vi "RFSoC_test.vi"() -> ()   [LabVIEW 2019]
uses:
  Pulse Parameters.ctl
  RFSoC Driver.lvclass
  C:/GitHub/NHMFL_Core/Libraries/Instruments/RFSoC/2019/GitHub/NHMFL_Core/Libraries/Instruments/Pulse Driver/Pulse Driver.lvclass
  RFSoC Driver.lvclass/RFSoC Driver.ctl
  Pulse Driver/Pulse Driver.lvclass/Pulse Driver.ctl
  Utilities/Output Value/Output Value.lvclass
  C:/GitHub/NHMFL_Core/Libraries/Instruments/RFSoC/2019/GitHub/NHMFL_Core/Libraries/Instruments/Results/Acquired Result/Acquired Result.lvclass
  Write address.vi
  Pulse Driver/Write Samples per read.vi
  Pulse Driver/Write Binary sample width.vi
  Write Mixer.vi
panel:
  in  "Mixer":enum16{"Real", "I/Q"}(ring)=enum."I/Q"
  in  "Samples per read":i32=8192
  in  "Tab Control":enum32{"Page 1", "Page 2"}(tab)
  in  "Send Button":bool
  out "Manual responce":string
  in  "Manual command":string
  in  "Initial commands SSR":string[](array[string])=["SetMemType 0", "SetBitstream 3", "MultiBand 0 0 0x1 0x2 0x1", "MultiBand 0 0 0x2 0x2 0x2", "SetMixerSettings 0 0 0 0.000000 0.000000 2 1 16 4 0", "UpdateEvent 0 0 0 1", "SetupFIFO 0 0 0", "SetDecimationFactor 0 0 1", "SetFabClkOutDiv 0 0 2", "IntrClr 0 0 0 0xFFFFFFFF", "SetupFIFO 0 0 1"]
  in  "Initial commands":string[](array[string])=["SetBitstream 1", "MultiBand 0 0 0x1 0x2 0x1", "MultiBand 0 0 0x2 0x2 0x2", "SetMixerSettings 0 0 0 -190.000000 0.000000 2 2 0 3 0", "UpdateEvent 0 0 0 1", "SetupFIFO 0 0 0", "SetDecimationFactor 0 0 1", "SetFabClkOutDiv 0 0 2", "IntrClr 0 0 0 0xFFFFFFFF", "SetupFIFO 0 0 1"]
  out "Responce":string[](array[string])
  out "Record responce":string[](array[string])
  in  "Generate commands 1":string[](array[string])=["LocalMemInfo 1", "LocalMemTrigger 1 0 0 0x0000"]
  in  "Generate commands 2":string[](array[string])=["SetLocalMemSample 1 1 3 8192", "LocalMemTrigger 1 1 0 0x0080", "LocalMemInfo 1"]
  out "Waveform Graph":cluster{dbl, dbl, dbl[][]}(graph)
  in  "Pulse Parameters":T1={"clock rate"=6389760000.0, "Frequency"=217000000.0, "NWaves"=75, "standard deviation"=0.1, "Amplitude"=30000.0, "Mode"=enum."Pulse"} {"Frequency" format="%#_6pHz"; "clock rate" format="%#_6pHz"}
  in  "Generate Button":bool
  in  "Output frequency":dbl=2000000.0 format="%#_6pHz"
  in  "Record  Button":bool
  out "FW Version":string
  in  "Stop Button":bool
  in  "address":string="192.168.1.3"
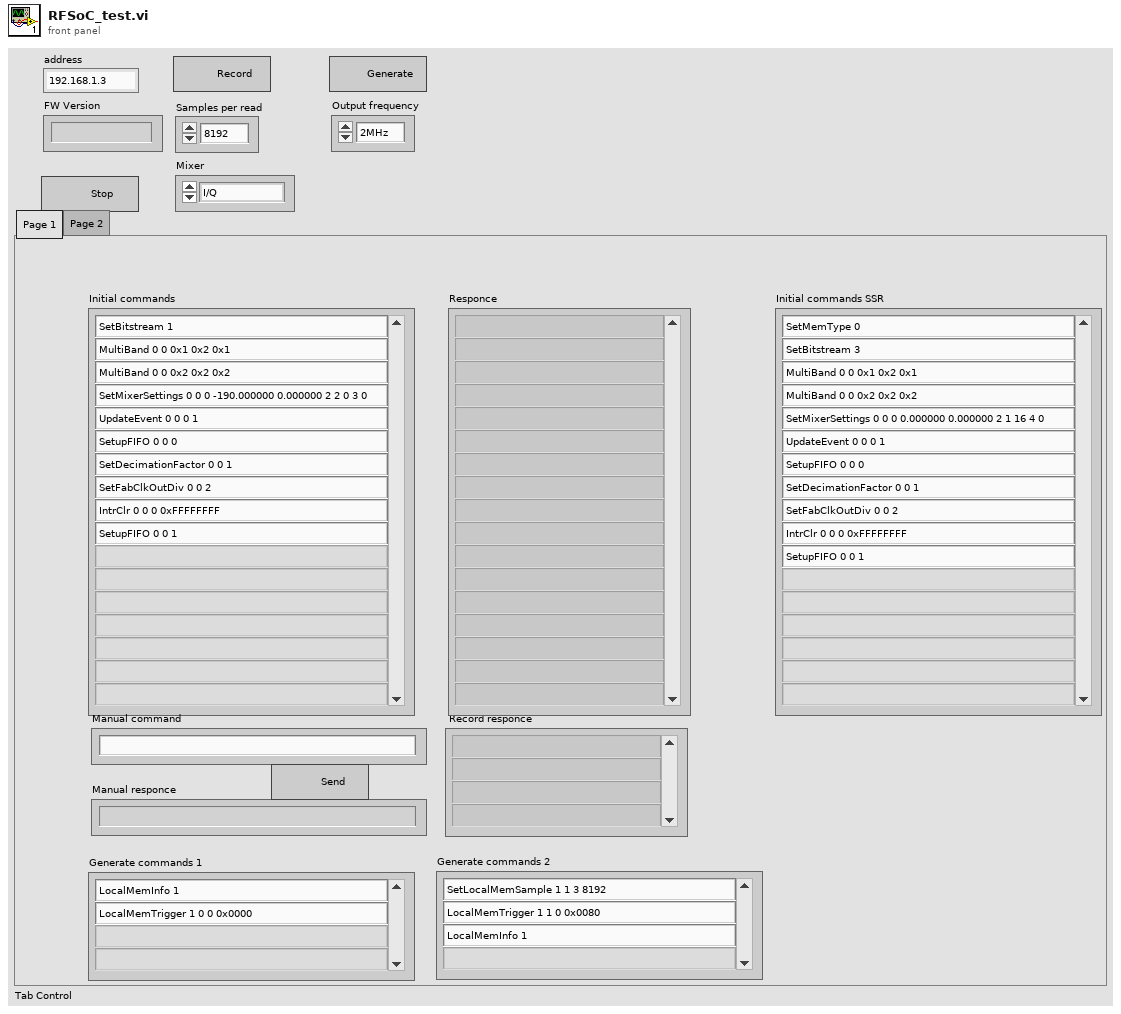
[diagram p1: front panel]
types:
  T1 = typedef "Pulse Parameters.ctl" = cluster{"clock rate":dbl, "Frequency":dbl, "NWaves":i32, "standard deviation":dbl, "Amplitude":dbl, "Mode":enum16{"Sine", "Pulse"}}
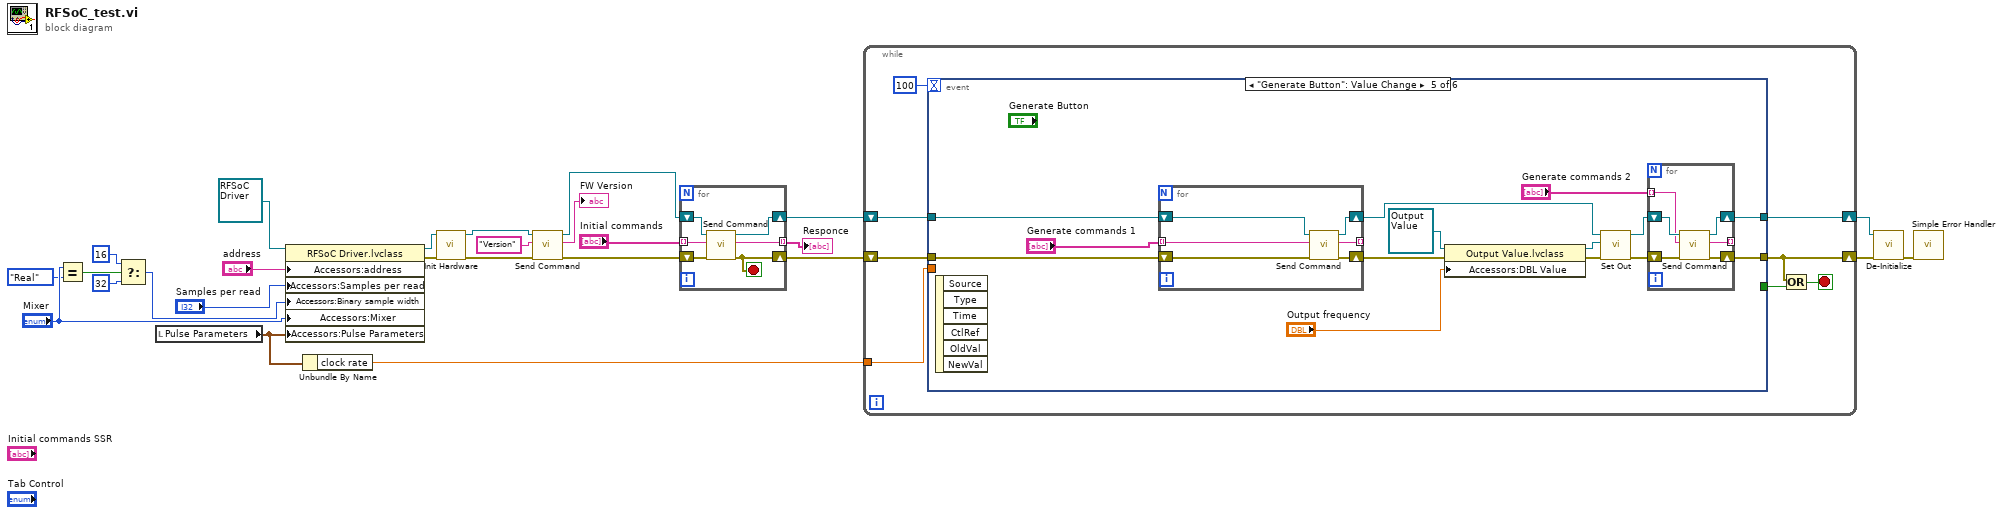
[diagram p0: block diagram]
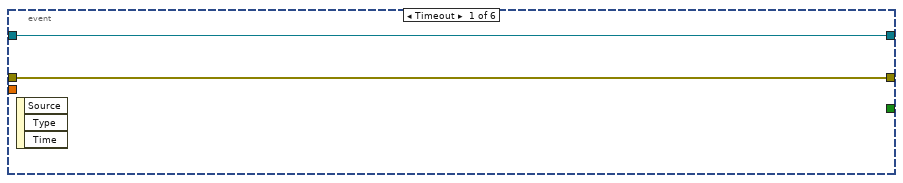
[diagram p2: hidden frame]
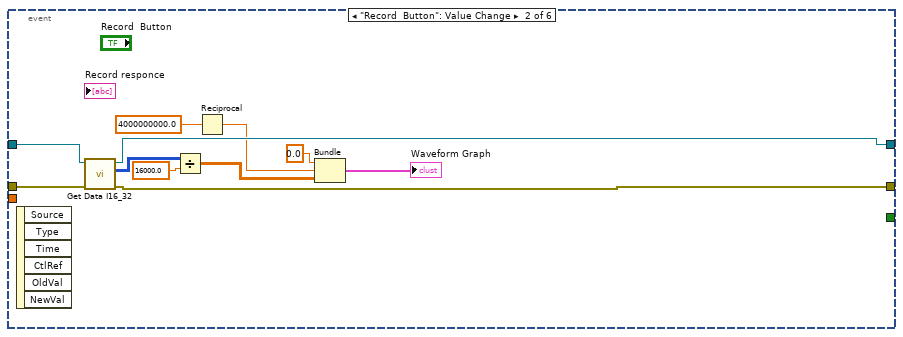
[diagram p3: hidden frame]
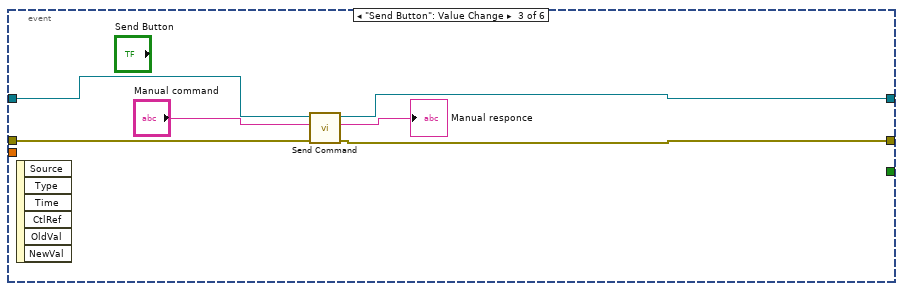
[diagram p4: hidden frame]
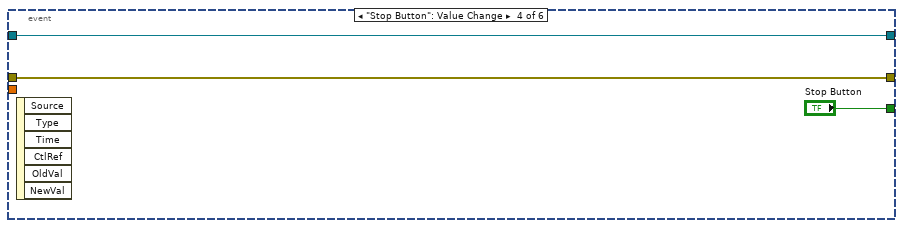
[diagram p5: hidden frame]
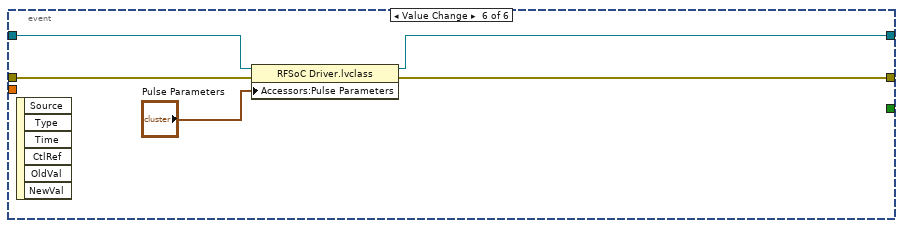
[diagram p6: hidden frame]
diagram:
  n1 = Equal?(x="Mixer", y=enum16{"Real", "I/Q"}."Real" ("Mixer")) -> (x = y?=w8:bool)
  n2 = Select(t=16 ("Binary sample width"), s=w8, f=32 ("Binary sample width")) -> (s? t:f=w4:i32)
  n3 = local read "Pulse Parameters"() -> (w2:T1)
  n4 = property class="RFSoC Driver.lvclass"(reference=refnum<class "RFSoC Driver.lvclass"> refnum ("RFSoC Driver.lvclass"), "Accessors:address"="address", "Accessors:Samples per read"="Samples per read", "Accessors:Binary sample width"=w4, "Accessors:Mixer"="Mixer", "Accessors:Pulse Parameters"=w2) -> (reference out=w18:refnum<class "RFSoC Driver.lvclass">, error out=w3:errorcluster)  [unwired: 1 in]
  n5 = Unbundle By Name(w2) -> ("clock rate"=w1:dbl)
  n6 = call-dynamic "Init Hardware.vi"("error in (no error)"=w3, "RFSoC Driver in"=w18) -> ("error out"=w24:errorcluster, "RFSoC Driver out"=w25:refnum<class "RFSoC Driver.lvclass">)  [unwired: 8 in]
  n7 = call-dynamic "Send Command.vi"("error in (no error)"=w24, "Command"="Version", "RFSoC Driver in"=w25) -> ("error out"=w15:errorcluster, "Responce"=→"FW Version":string, "RFSoC Driver out"=w16:refnum<class "RFSoC Driver.lvclass">)  [unwired: 6 in]
  n8 = for {
    tunnel: "Initial commands" -> [w31] mode=indexing
    shift-right: [w29] -> w11
    shift-left: w16 -> [w32]
    shift-right: [w27] -> w12
    shift-left: w15 -> [w30]
    tunnel: [w28] -> w13 mode=indexing
    stop <- w27 stop-if-true
    n9 = call-dynamic "Send Command.vi"("error in (no error)"=w30, "Command"=w31, "RFSoC Driver in"=w32) -> ("error out"=w27:errorcluster, "Responce"=w28:string, "RFSoC Driver out"=w29:refnum<class "RFSoC Driver.lvclass">)  [unwired: 6 in]
  }
  "Responce" <- w13
  n10 = while {
    shift-right: [w39] -> w20
    shift-left: w11 -> [w40]
    shift-right: [w37] -> w21
    shift-left: w12 -> [w38]
    tunnel: w1 -> [w33]
    stop <- w35 stop-if-true
    n11 = event shown="[4] \"Generate Button\": Value Change" {
      selector: _ -> [_ _ _ _ _ _]
      dyn-events: _ -> [_ _ _ _ _ _]
      timeout: 100 -> [_ _ _ _ _ _]
      tunnel: [_ _ _ "Stop Button" _ _] -> w36
      tunnel: w40 -> [w42 w53 w59 w61 w71 w93]
      tunnel: [w42 w51 w55 w61 w66 w89] -> w39
      tunnel: w38 -> [w41 w52 w58 w60 w69 w91]
      tunnel: [w41 w50 w54 w60 w65 w90] -> w37
      tunnel: w33 -> [_ _ _ _ _ _]
      event Timeout {
        n12 = event-data() -> ()  [unwired: 1 in, 3 out]
      }
      event "Record  Button": Value Change {
        n13 = event-data() -> ()  [unwired: 1 in, 6 out]
        n14 = call-dynamic "Get Data I16_32.vi"("error in (no error)"=w52, "RFSoC Driver in"=w53) -> ("error out"=w50:errorcluster, "I16 data out"=w47:i16[][], "RFSoC Driver out"=w51:refnum<class "RFSoC Driver.lvclass">)  [unwired: 4 in, 3 out]
        n15 = Divide(x=w47, y=16000.0) -> (x/y=w45:dbl[][])
        n16 = Reciprocal(x=4000000000.0) -> (1/x=w48:dbl)
        n17 = Bundle(0.0, w48, w45) -> (→"Waveform Graph":cluster{dbl, dbl, dbl[][]})  [unwired: 1 in]
      }
      event "Send Button": Value Change {
        n18 = event-data() -> ()  [unwired: 1 in, 6 out]
        n19 = call-dynamic "Send Command.vi"("error in (no error)"=w58, "Command"="Manual command", "RFSoC Driver in"=w59) -> ("error out"=w54:errorcluster, "Responce"=→"Manual responce":string, "RFSoC Driver out"=w55:refnum<class "RFSoC Driver.lvclass">)  [unwired: 6 in]
      }
      event "Stop Button": Value Change {
        n20 = event-data() -> ()  [unwired: 1 in, 6 out]
      }
      event "Generate Button": Value Change {
        n21 = event-data() -> ()  [unwired: 1 in, 6 out]
        n22 = for {
          shift-right: [w85] -> w70
          shift-left: w71 -> [w88]
          shift-right: [w84] -> w68
          shift-left: w69 -> [w87]
          tunnel: "Generate commands 1" -> [w86] mode=indexing
          tunnel: [w83] -> _ mode=indexing
          n23 = call-dynamic "Send Command.vi"("error in (no error)"=w87, "Command"=w86, "RFSoC Driver in"=w88) -> ("error out"=w84:errorcluster, "Responce"=w83:string, "RFSoC Driver out"=w85:refnum<class "RFSoC Driver.lvclass">)  [unwired: 6 in]
        }
        n24 = property class="Output Value.lvclass"(reference=refnum<class "Output Value.lvclass"> refnum ("Output value"), error in=w68, "Accessors:DBL Value"="Output frequency") -> (reference out=w74:refnum<class "Output Value.lvclass">, error out=w76:errorcluster)
        n25 = call-dynamic "Set Out.vi"("error in (no error)"=w76, "Output value"=w74, "RFSoC Driver in"=w70) -> ("error out"=w64:errorcluster, "RFSoC Driver out"=w67:refnum<class "RFSoC Driver.lvclass">)  [unwired: 7 in]
        n26 = for {
          shift-right: [w80] -> w66
          shift-left: w67 -> [w82]
          shift-right: [w79] -> w65
          shift-left: w64 -> [w81]
          tunnel: [w78] -> _ mode=indexing
          tunnel: "Generate commands 2" -> [w77] mode=indexing
          n27 = call-dynamic "Send Command.vi"("error in (no error)"=w81, "Command"=w77, "RFSoC Driver in"=w82) -> ("error out"=w79:errorcluster, "Responce"=w78:string, "RFSoC Driver out"=w80:refnum<class "RFSoC Driver.lvclass">)  [unwired: 6 in]
        }
      }
      event Value Change {
        n28 = event-data() -> ()  [unwired: 1 in, 6 out]
        n29 = property class="RFSoC Driver.lvclass"(reference=w93, error in=w91, "Accessors:Pulse Parameters"="Pulse Parameters") -> (reference out=w89:refnum<class "RFSoC Driver.lvclass">, error out=w90:errorcluster)
      }
    }
    n30 = Or(x=w37, y=w36) -> (x .or. y?=w35:bool)
  }
  n31 = call-dynamic "De-Initialize.vi"("error in (no error)"=w21, "RFSoC Driver in"=w20) -> ("error out"=w19:errorcluster)  [unwired: 8 in, 1 out]
  n32 = call <vilib>:"Simple Error Handler.vi"("error in (no error)"=w19) -> ()  [unwired: 4 in, 5 out]
